vi "readValues.vi"(7 "isChangingSwitchHeaterState":bool, 8 "Error In":errorcluster, 9 "AMI_Cluster in":T1, 10 "VISA resource name Y axis":refnum<visa-resource-name>, 11 "VISA resource nanme Z axis":refnum<visa-resource-name>) -> (0 "Error Out":errorcluster, 1 "AMI_Cluster out":T1, 2 "VISA resource name out Y axis":refnum<visa-resource-name>, 3 "VISA resource name out Z axis":refnum<visa-resource-name>)   [LabVIEW 2019]
uses:
  Monitor Communication/AMI/AMI_cluster.ctl
  Global/Global Variables/Data_Display_global.vi
panel:
  # "AMI-Cluster"
  # "AMI-Cluster"
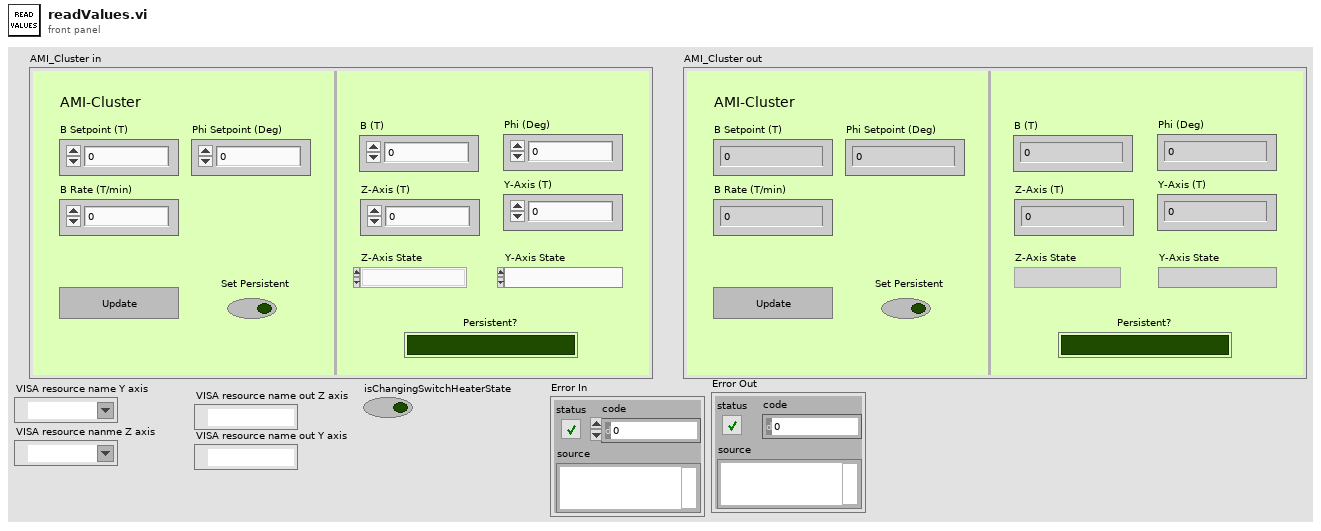
[diagram p1: front panel]
types:
  T1 = typedef "AMI_cluster.ctl" = cluster{"Set Persistent":bool, "B (T)":dbl, "B Setpoint (T)":dbl, "Phi (Deg)":dbl, "Phi Setpoint (Deg)":dbl, "B Rate (T/min)":dbl, "Y-Axis (T)":dbl, "Z-Axis (T)":dbl, "Z-Axis State":enum16{"", "RAMPING", "HOLDING", "PAUSED", "MANUAL UP", "MANUAL DOWN", "ZEROING CURRENT", "QUENCH DETECTED", "AT ZERO", "HEATING SWITCH", "COOLING SWITCH", "EXTERNAL RAMPDOWN"}, "Y-Axis State":enum16{"", "RAMPING", "HOLDING", "PAUSED", "MANUAL UP", "MANUAL DOWN", "ZEROING CURRENT", "QUENCH DETECTED", "AT ZERO", "HEATING SWITCH", "COOLING SWITCH", "EXTERNAL RAMPDOWN"}, "Update":bool, "Persistent?":bool}
  T2 = cluster{"error":bool, "code":i32, "source":string}
  T3 = enum16{"", "RAMPING", "HOLDING", "PAUSED", "MANUAL UP", "MANUAL DOWN", "ZEROING CURRENT", "QUENCH DETECTED", "AT ZERO", "HEATING SWITCH", "COOLING SWITCH", "EXTERNAL RAMPDOWN"}
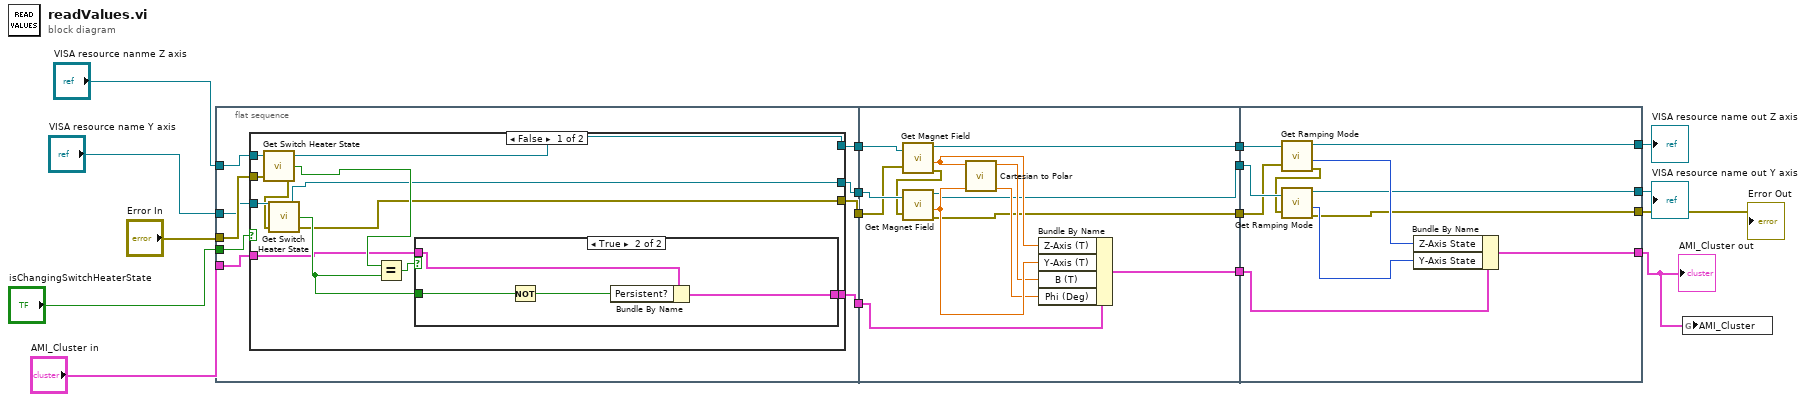
[diagram p0: block diagram]
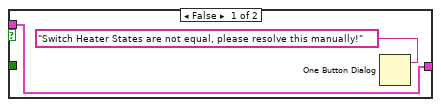
[diagram p2: hidden frame]
diagram:
  n1 = flat-sequence {
    tunnel: "Error In" -> [w24]
    tunnel: "VISA resource nanme Z axis" -> [w26]
    tunnel: [w19] -> w17
    tunnel: [w25] -> w16
    tunnel: [w23] -> w15
    tunnel: [w22] -> w14
    tunnel: "AMI_Cluster in" -> [w21]
    tunnel: "VISA resource name Y axis" -> [w20]
    tunnel: "isChangingSwitchHeaterState" -> [w18]
    tunnel: w17 -> [w55]
    tunnel: w16 -> [w57]
    tunnel: w15 -> [w56]
    tunnel: [w54] -> w13
    tunnel: [w53] -> w12
    tunnel: [w49] -> w11
    tunnel: w14 -> [w52]
    tunnel: [w51] -> w10
    tunnel: w13 -> [w69]
    tunnel: w12 -> [w70]
    tunnel: w11 -> [w64]
    tunnel: [w68] -> w5
    tunnel: [w67] -> w4
    tunnel: [w62] -> w3
    tunnel: w10 -> [w66]
    tunnel: [w65] -> w2
    frame #0 {
      n2 = case shown="False" w18 {
        tunnel: w26 -> [w35 w48]
        tunnel: [w34 w48] -> w25
        tunnel: w24 -> [w33 w47]
        tunnel: [w32 w46] -> w23
        tunnel: [w31 w45] -> w22
        tunnel: w21 -> [w30 w45]
        tunnel: w20 -> [w29 w46]
        tunnel: [w27 w47] -> w19
        frame False {
          n3 = call "Get Switch Heater State.vi"("error in"=w33, "VISA resource name"=w35) -> ("error out"=w28:T2, "Switch Heater state"=w37:bool, "VISA resource name out"=w34:refnum<visa-resource-name>)  [unwired: 1 in]
          n4 = call "Get Switch Heater State.vi"("error in"=w28, "VISA resource name"=w29) -> ("error out"=w27:T2, "Switch Heater state"=w38:bool, "VISA resource name out"=w32:refnum<visa-resource-name>)  [unwired: 1 in]
          n5 = Equal?(x=w37, y=w38) -> (x = y?=w36:bool)
          n6 = case shown="True" w36 {
            tunnel: w38 -> [_ w43]
            tunnel: [w39 w42] -> w31
            tunnel: w30 -> [w39 w41]
            frame False {
              n7 = One Button Dialog(message="Switch Heater States are not equal, please resolve this manually!") -> ()  [unwired: 1 in, 1 out]
            }
            frame True {
              n8 = Not(x=w43) -> (.not. x?=w44:bool)
              n9 = Bundle By Name(cluster=w41, "Persistent?"=w44) -> (w42:T1)
            }
          }
        }
        frame True {
        }
      }
    }
    frame #1 {
      n10 = call "Get Magnet Field.vi"("VISA resource name"=w57, "error in"=w55) -> ("VISA resource name out"=w54:refnum<visa-resource-name>, "Magnet Field (kG)"=w60:dbl, "error out"=w50:T2)  [unwired: 1 out]
      n11 = call "Get Magnet Field.vi"("VISA resource name"=w56, "error in"=w50) -> ("VISA resource name out"=w53:refnum<visa-resource-name>, "Magnet Field (kG)"=w61:dbl, "error out"=w49:T2)  [unwired: 1 out]
      n12 = call "Cartesian to Polar.vi"("Y"=w61, "Z"=w60) -> ("Phi"=w58:dbl, "B"=w59:dbl)  [unwired: 8 in]
      n13 = Bundle By Name(cluster=w52, "Z-Axis (T)"=w60, "Y-Axis (T)"=w61, "B (T)"=w59, "Phi (Deg)"=w58) -> (w51:T1)
    }
    frame #2 {
      n14 = call "Get Ramping Mode.vi"("VISA resource name"=w69, "error in"=w64) -> ("VISA resource name out"=w68:refnum<visa-resource-name>, "Ramping Mode"=w71:T3, "error out"=w63:T2)  [unwired: 1 out]
      n15 = call "Get Ramping Mode.vi"("VISA resource name"=w70, "error in"=w63) -> ("VISA resource name out"=w67:refnum<visa-resource-name>, "Ramping Mode"=w72:T3, "error out"=w62:T2)  [unwired: 1 out]
      n16 = Bundle By Name(cluster=w66, "Z-Axis State"=w71, "Y-Axis State"=w72) -> (w65:T1)
    }
  }
  n17 = global write "Data_Display_global.vi" "AMI_Cluster"(w2) -> ()
  "AMI_Cluster out" <- w2
  "VISA resource name out Z axis" <- w5
  "VISA resource name out Y axis" <- w4
  "Error Out" <- w3
